vi "UHR-Fleezers Control (host) - 10.6.vi"() -> ()   [LabVIEW 2011] (continued)
              frame False {
              }
              frame True {
                n360 = property on="Sample Channel\nFlow" class="Bool (strict)"("Val(Sgnl)"=TRUE ("Stage Moving")) -> ()  [unwired: 2 in, 2 out]
              }
            }
            n361 = local write "Fl. Triggered..."(w574) -> ()
            n362 = local write "Tether"(w574) -> ()
            n363 = property on="Green Laser ON/Interlacing" class="Bool (strict)"("Val(Sgnl)"=w574) -> ()  [unwired: 2 in, 2 out]
            n364 = property on="Trap Pos. FB ON" class="Bool (strict)"("Val(Sgnl)"=w574) -> ()  [unwired: 2 in, 2 out]
            n365 = property on="Trap Trig. Fl." class="Bool (strict)"("Val(Sgnl)"=w574) -> ()  [unwired: 2 in, 2 out]
            n366 = property on="Dip for Protein" class="Bool (strict)"("Val(Sgnl)"=w574) -> ()  [unwired: 2 in, 2 out]
            n367 = property on="Pause dwell" class="Bool (strict)"("Val(Sgnl)"=w574) -> ()  [unwired: 2 in, 2 out]
          }
          frame #2 {
            n368 = property on="Trap Pos. FB Offset Factor" class="DigNum (strict)"("Val(Sgnl)"=i64 0 ("Value (Signaling)")) -> ()  [unwired: 2 in, 2 out]
          }
          frame #3 {
            n369 = local read "Saved Stage Positions"() -> (w583:dbl[][])
            n370 = local write "Stage Moving"(TRUE ("Stage Moving")) -> ()
            n371 = Array Subset(array=w583, index (row)=3 ("index"), length (row)=1 ("length"), index (col)=1 ("index"), length (col)=3 ("length")) -> (w588:dbl[][])
            n372 = Reshape Array(w588, 3 ("dimension size")) -> (w586:dbl[])
            n373 = Array To Cluster(array=w586) -> (cluster=w585:cluster{"[0]":dbl, "[1]":dbl, "[2]":dbl})
            n374 = call "Set Stage Position.vi"("Position"=w585, "error in"=w581, "VISA resource name in"=w582) -> ()  [unwired: 3 out]
          }
          frame #4 {
            w593 = FALSE ("Value (Signaling)")
            n375 = case shown="True" w592 {
              frame False {
              }
              frame True {
                n376 = property on="Sample Channel\nFlow" class="Bool (strict)"("Val(Sgnl)"=FALSE ("Stage Moving")) -> ()  [unwired: 2 in, 2 out]
              }
            }
            n377 = property on="Trap 1 (ON/OFF)" class="Bool (strict)"("Val(Sgnl)"=w593) -> ()  [unwired: 2 in, 2 out]
            n378 = property on="Trap 2 (ON/OFF)" class="Bool (strict)"("Val(Sgnl)"=w593) -> ()  [unwired: 2 in, 2 out]
            n379 = call <vilib>:"Beep.vi"() -> ()  [unwired: 3 in, 9 out]
          }
          frame #5 {
            n380 = property on="Move Cap. 2 (ADig Top)" class="Bool (strict)"("Val(Sgnl)"=TRUE ("Value (Signaling)")) -> ()  [unwired: 2 in, 2 out]
            n381 = property on="Tab Control" class="TabCtl (strict)"("Val(Sgnl)"=T4."Status" ("Value (Signaling)")) -> ()  [unwired: 2 in, 2 out]
          }
        }
      }
      event "Dip for Protein": Value Change {
        n382 = event-data() -> ()  [unwired: 1 in, 5 out]
        n383 = case shown="True" "Dip for Protein" {
          tunnel: w599 -> [_ w601]
          tunnel: w598 -> [_ w600]
          frame False {
          }
          frame True {
            n384 = while {
              tunnel: w601 -> [w612]
              tunnel: w600 -> [w611]
              i -> [w606]
              stop <- w608 stop-if-true
              n385 = Increment(x=w606) -> (x+1=→"Dip #":i32)
              n386 = flat-sequence {
                tunnel: w611 -> [w623]
                tunnel: w612 -> [w624]
                tunnel: [w624] -> w616
                tunnel: [w623] -> w615
                tunnel: [w617] -> w602
                tunnel: [w629] -> w610
                tunnel: [w630] -> w609
                tunnel: w616 -> [w631]
                tunnel: w615 -> [w632]
                tunnel: [w627] -> w603
                tunnel: w602 -> [w627]
                tunnel: [w640] -> w614
                tunnel: w610 -> [w640]
                tunnel: [w639] -> w613
                tunnel: w609 -> [w639]
                tunnel: [w636] -> w607
                tunnel: [w635] -> w604
                tunnel: w603 -> [w635]
                tunnel: w613 -> [w660]
                tunnel: w614 -> [w661]
                tunnel: w607 -> [w662]
                tunnel: w604 -> [w659]
                tunnel: [w718] -> w608
                frame #0 {
                  n387 = local read "Trap Pos. FB ON"() -> (w617:bool)
                  n388 = Compound Arithmetic op=AND("Flow ON\nduring dip?", "FB OFF when \nflow ON", w617) -> (w618:bool)
                  n389 = case shown="True" "Move trap \nbefore dip move?" {
                    frame False {
                    }
                    frame True {
                      n390 = property on="Trap Delta (MHz)" class="DigNum (strict)"("Val(Sgnl)"="Dipping Delta (MHz)") -> ()  [unwired: 2 in, 2 out]
                    }
                  }
                  n391 = property on="Green Laser ON/Interlacing" class="Bool (strict)"("Val(Sgnl)"="Green ON\nbefore dip?") -> ()  [unwired: 2 in, 2 out]
                  n392 = property on="Sample Channel\nFlow" class="Bool (strict)"("Val(Sgnl)"="Flow ON\nduring dip?") -> ()  [unwired: 2 in, 2 out]
                  n393 = case shown="True" w618 {
                    frame False {
                    }
                    frame True {
                      n394 = property on="Trap Pos. FB ON" class="Bool (strict)"("Val(Sgnl)"=FALSE ("Value (Signaling)")) -> ()  [unwired: 2 in, 2 out]
                    }
                  }
                }
                frame #1 {
                  n395 = local read "Saved Stage Positions"() -> (w634:dbl[][])
                  n396 = local write "Cancel dwell"(FALSE ("Cancel dwell")) -> ()
                  n397 = call "move to saved stage position.vi"("error in"=w632, "Stage VISA resource name in"=w631, "Position"="Dip Stage \nPosition", "Saved Stage Positions"=w634) -> ("VISA resource name out"=w629:refnum<visa-resource-name>, "error out"=w630:errorcluster)
                }
                frame #2 {
                  n398 = node-c288() -> (w638:T21)  [unwired: 4 in]
                  n399 = timed-loop {
                    timing: w638 -> [_]
                    timing-out: [_] -> w637
                    tunnel: [w644] -> w636
                    i -> [w641]
                    stop <- w645 stop-if-true
                    n400 = node-c288() -> ()  [unwired: 1 in, 1 out]
                    n401 = Greater Or Equal?(x=w641, y="Dip Duration (s)") -> (x >= y?=w653:bool)
                    n402 = local read "Dip for Protein"() -> (w646:bool)
                    n403 = local read "Dump Beads"() -> (w643:bool)
                    n404 = local read "Cancel dwell"() -> (w652:bool)
                    n405 = local read "Pause dwell"() -> (w649:bool)
                    n406 = Not(x=w646) -> (.not. x?=w651:bool)
                    n407 = Compound Arithmetic op=OR(w652, w653, w651) -> (w650:bool)
                    n408 = Select(t=FALSE, s=w649, f=w650) -> (s? t:f=w647:bool)
                    n409 = Not(x=w643) -> (.not. x?=w642:bool)
                    n410 = node-c288() -> ()  [unwired: 1 in, 1 out]
                    n411 = And(x=w646, y=w642) -> (x .and. y?=w644:bool)
                    n412 = Or(x=w647, y=w643) -> (x .or. y?=w645:bool)
                    "Dip Time (s)" <- w641
                  }
                  n413 = node-c288(w637) -> ()  [unwired: 1 out]
                }
                frame #3 {
                  n414 = case shown="True" w662 {
                    tunnel: w661 -> [_ w667]
                    tunnel: w660 -> [_ w666]
                    tunnel: w659 -> [_ w663]
                    frame False {
                    }
                    frame True {
                      n415 = flat-sequence {
                        tunnel: w666 -> [w671]
                        tunnel: w667 -> [w672]
                        tunnel: [w672] -> w665
                        tunnel: [w671] -> w664
                        tunnel: w663 -> [w668]
                        tunnel: w665 -> [w682]
                        tunnel: w664 -> [w681]
                        tunnel: w663 -> [w690]
                        frame #0 {
                          n416 = local read "Sample Channel\nFlow"() -> (w670:bool)
                          n417 = case shown="False" w670 {
                            tunnel: "Flow ON \nduring return\nfrom dip?" -> [w673 w676]
                            tunnel: w668 -> [_ w675]
                            frame False {
                              n418 = case shown="True" w673 {
                                frame False {
                                }
                                frame True {
                                n419 = property on="Sample Channel\nFlow" class="Bool (strict)"("Val(Sgnl)"=TRUE ("Value (Signaling)")) -> ()  [unwired: 2 in, 2 out]
                                }
                              }
                            }
                            frame True {
                              n420 = case shown="False" w676 {
                                tunnel: w675 -> [w677 _]
                                frame False {
                                n421 = property on="Trap Pos. FB ON" class="Bool (strict)"("Val(Sgnl)"=w677) -> ()  [unwired: 2 in, 2 out]
                                n422 = property on="Sample Channel\nFlow" class="Bool (strict)"("Val(Sgnl)"=FALSE ("Value (Signaling)")) -> ()  [unwired: 2 in, 2 out]
                                }
                                frame True {
                                }
                              }
                            }
                          }
                        }
                        frame #1 {
                          # "For turning on green laser before stage reaches lower spot"
                          n423 = case shown="True" "Green ON\nafter start\nreturn?" {
                            frame False {
                            }
                            frame True {
                              n424 = flat-sequence {
                                frame #0 {
                                n425 = Multiply(x="Green delay after \nstart return (s)", y=1000.0) -> (x*y=w687:dbl)
                                n426 = Wait (ms)(milliseconds to wait=w687) -> ()  [unwired: 1 out]
                                }
                                frame #1 {
                                n427 = property on="Green Laser ON/Interlacing" class="Bool (strict)"("Val(Sgnl)"=TRUE ("Value (Signaling)")) -> ()  [unwired: 2 in, 2 out]
                                }
                              }
                            }
                          }
                          n428 = local read "Saved Stage Positions"() -> (w685:dbl[][])
                          n429 = local write "Cancel dwell"(FALSE ("Cancel dwell")) -> ()
                          n430 = call "move to saved stage position.vi"("error in"=w681, "Stage VISA resource name in"=w682, "Position"="Return Stage \nPosition", "Saved Stage Positions"=w685) -> ("error out"=w683:errorcluster)  [unwired: 1 out]
                          n431 = local write "Stage Control Serial Error"(w683) -> ()
                        }
                        frame #2 {
                          n432 = property on="Trap Pos. FB ON" class="Bool (strict)"("Val(Sgnl)"=w690) -> ()  [unwired: 2 in, 2 out]
                          n433 = case shown="True" "Green ON \nafter return?" {
                            frame False {
                            }
                            frame True {
                              n434 = property on="Green Laser ON/Interlacing" class="Bool (strict)"("Val(Sgnl)"=TRUE ("Value (Signaling)")) -> ()  [unwired: 2 in, 2 out]
                            }
                          }
                          n435 = case shown="True" "Move trap after return?" {
                            frame False {
                            }
                            frame True {
                              n436 = property on="Trap Delta (MHz)" class="DigNum (strict)"("Val(Sgnl)"="Dip Trap Delta 2 (MHz)") -> ()  [unwired: 2 in, 2 out]
                            }
                          }
                          n437 = case shown="True" "Save data after return?" {
                            frame False {
                            }
                            frame True {
                              n438 = property on="Start Saving" class="Bool (strict)"("Val(Sgnl)"=TRUE ("Value (Signaling)")) -> ()  [unwired: 2 in, 2 out]
                            }
                          }
                          n439 = property on="Sample Channel\nFlow" class="Bool (strict)"("Val(Sgnl)"="Flow ON\nduring daq?") -> ()  [unwired: 2 in, 2 out]
                        }
                        frame #3 {
                          n440 = node-c288() -> (w699:T21)  [unwired: 4 in]
                          n441 = timed-loop {
                            timing: w699 -> [_]
                            timing-out: [_] -> w698
                            i -> [w700]
                            stop <- w702 stop-if-true
                            n442 = node-c288() -> ()  [unwired: 1 in, 1 out]
                            n443 = local read "Dump Beads"() -> (w701:bool)
                            n444 = Greater Or Equal?(x=w700, y="Dwell Duration (s)") -> (x >= y?=w707:bool)
                            n445 = local read "Dip for Protein"() -> (w704:bool)
                            n446 = Not(x=w704) -> (.not. x?=w703:bool)
                            n447 = Compound Arithmetic op=OR(w707, "Cancel dwell", w703) -> (w706:bool)
                            n448 = node-c288() -> ()  [unwired: 1 in, 1 out]
                            n449 = Select(t=FALSE, s="Pause dwell", f=w706) -> (s? t:f=w709:bool)
                            n450 = Or(x=w709, y=w701) -> (x .or. y?=w702:bool)
                            "Dwell Time (s)" <- w700
                          }
                          n451 = node-c288(w698) -> ()  [unwired: 1 out]
                        }
                      }
                    }
                  }
                }
                frame #4 {
                  n452 = local read "Dip for Protein"() -> (w719:bool)
                  n453 = local read "Dump Beads"() -> (w716:bool)
                  n454 = local write "Cancel dwell"(FALSE ("Cancel dwell")) -> ()
                  n455 = Not(x=w719) -> (.not. x?=w720:bool)
                  n456 = Not(x="Cont. Repeat Dipping?") -> (.not. x?=w722:bool)
                  n457 = Compound Arithmetic op=OR(w720, w722, w716) -> (w718:bool)
                }
              }
            }
          }
        }
      }
      event "Profile": Value Change {
        n458 = event-data() -> ()  [unwired: 1 in, 5 out]
        n459 = flat-sequence {
          tunnel: w731 -> [w734]
          tunnel: w730 -> [w742]
          tunnel: [w736] -> w729
          tunnel: [w735] -> w728
          tunnel: [w733] -> w726
          tunnel: [w732] -> w723
          tunnel: w729 -> [w749]
          tunnel: w728 -> [w748]
          tunnel: [w746] -> w727
          tunnel: w726 -> [w747]
          tunnel: [w745] -> w725
          tunnel: [w744] -> w724
          tunnel: w723 -> [w744]
          tunnel: w727 -> [w753]
          tunnel: w725 -> [w752]
          tunnel: w724 -> [w751]
          frame #0 {
            n460 = call "Read Stage Position.vi"("error in"=w742, "VISA resource name in"=w734) -> ("Current Position"=w732:cluster{dbl, dbl, dbl}, "error out"=w735:errorcluster, "VISA resource name out"=w733:refnum<visa-resource-name>)  [unwired: 1 out]
            "Current Position" <- w732
            n461 = local write "Stage Control Serial Error"(w735) -> ()
            n462 = Unbundle(w732) -> (w739:dbl, w741:dbl, w737:dbl)
            n463 = Add(x=w741, y="Y change (mm)") -> (x+y=w738:dbl)
            n464 = Bundle(w739, w738, w737) -> (w736:cluster{dbl, dbl, dbl})  [unwired: 1 in]
          }
          frame #1 {
            # "move to new position and start saving"
            n465 = local write "Stage Moving"(TRUE ("Stage Moving")) -> ()
            n466 = local write "Start Saving"(TRUE ("Start Saving")) -> ()
            n467 = call "Set Stage Position.vi"("Position"=w749, "error in"=w748, "VISA resource name in"=w747) -> ("error out"=w745:errorcluster, "VISA resource name out"=w746:refnum<visa-resource-name>)  [unwired: 1 out]
          }
          frame #2 {
            # "go back to start"
            n468 = call "Set Stage Position.vi"("Position"=w751, "error in"=w752, "VISA resource name in"=w753) -> ()  [unwired: 3 out]
          }
          frame #3 {
            # "stop saving"
            n469 = local write "Stop Saving"(TRUE ("Stop Saving")) -> ()
            n470 = local write "Stage Moving"(FALSE ("Stage Moving")) -> ()
          }
        }
      }
      event "Move to Position 1", "Move to Position 2", "Move to Position 3", "Move to Position 4", "Move to Position 5", "Lower Ch. Cap.": Value Change {
        n471 = event-data() -> ()  [unwired: 1 in, 5 out]
        n472 = Or(x="Move to Position 5", y="Lower Ch. Cap.") -> (x .or. y?=w759:bool)
        n473 = Build Array("Move to Position 1", "Move to Position 2", "Move to Position 3", "Move to Position 4", w759) -> (w762:bool[])
        n474 = Boolean Array To Number(Boolean array=w762) -> (number=w761:u32)
        n475 = Logarithm Base 2(1:w761) -> (0:w760:dbl)
        n476 = flat-sequence {
          tunnel: w760 -> [w771]
          tunnel: w757 -> [w769]
          tunnel: w756 -> [w768]
          frame #0 {
            n477 = local read "Saved Stage Positions"() -> (w779:dbl[][])
            n478 = Array Subset(array=w779, index (row)=w771, length (row)=1 ("length"), index (col)=1 ("index"), length (col)=3 ("length")) -> (w776:dbl[][])
            n479 = Reshape Array(w776, 3 ("dimension size")) -> (w774:dbl[])
            n480 = Array To Cluster(array=w774) -> (cluster=w773:cluster{"[0]":dbl, "[1]":dbl, "[2]":dbl})
            n481 = call "Set Stage Position.vi"("Position"=w773, "error in"=w768, "VISA resource name in"=w769) -> ("error out"=w772:errorcluster)  [unwired: 2 out]
            n482 = local write "Stage Moving"(TRUE ("Stage Moving")) -> ()
            n483 = local write "Stage Control Serial Error"(w772) -> ()
          }
          frame #1 {
            n484 = local write "Stage Moving"(FALSE ("Stage Moving")) -> ()
            n485 = call <vilib>:"Beep.vi"() -> ()  [unwired: 3 in, 9 out]
          }
        }
      }
      event "Got ADig bead": Value Change {
        n486 = event-data() -> ()  [unwired: 1 in, 5 out]
        n487 = flat-sequence {
          frame #0 {
            n488 = local read "Cap 1 Samp Flow ON"() -> (w783:bool)
            n489 = case shown="True" w783 {
              frame False {
              }
              frame True {
                n490 = property on="Sample Channel\nFlow" class="Bool (strict)"("Val(Sgnl)"=TRUE ("Value (Signaling)")) -> ()  [unwired: 2 in, 2 out]
              }
            }
          }
          frame #1 {
            n491 = property on="Inject Pump 3" class="Bool (strict)"("Val(Sgnl)"=FALSE ("Value (Signaling)")) -> ()  [unwired: 2 in, 2 out]
          }
          frame #2 {
            n492 = property on="Move Cap. 1 (DNA Bottom)" class="Bool (strict)"("Val(Sgnl)"=TRUE ("Value (Signaling)")) -> ()  [unwired: 2 in, 2 out]
          }
        }
      }
      event "Force FB Data\nScript": Value Change {
        n493 = event-data() -> ()  [unwired: 1 in, 5 out]
        n494 = flat-sequence {
          tunnel: w792 -> [w796]
          tunnel: w793 -> [w797]
          tunnel: [w797] -> w788
          tunnel: [w796] -> w787
          tunnel: w788 -> [w800]
          tunnel: w787 -> [w799]
          tunnel: ["Trap Trig Fl."] -> w789
          tunnel: [w825] -> w790
          tunnel: w789 -> [w825]
          tunnel: [w829] -> w791
          tunnel: w790 -> [w829]
          tunnel: w791 -> [w831]
          frame #0 {
            n495 = property on="Trap Delta (MHz)" class="DigNum (strict)"("Val(Sgnl)"="Trap Delta Before Moving") -> ()  [unwired: 2 in, 2 out]
          }
          frame #1 {
            n496 = local read "Saved Stage Positions"() -> (w802:dbl[][])
            n497 = local write "FB Trap Pos Offset"(0.0 ("FB Trap Pos Offset")) -> ()
            n498 = property on="Trap Pos. FB Offset Factor" class="DigNum (strict)"("Val(Sgnl)"=i64 0 ("Value (Signaling)")) -> ()  [unwired: 2 in, 2 out]
            n499 = local write "Stage Moving"(TRUE ("Stage Moving")) -> ()
            n500 = call "move to saved stage position.vi"("error in"=w799, "Stage VISA resource name in"=w800, "Position"="Stage Position To Establish FB", "Saved Stage Positions"=w802) -> ("error out"=w798:errorcluster)  [unwired: 1 out]
            n501 = local write "Stage Control Serial Error"(w798) -> ()
          }
          frame #2 {
            n502 = call <vilib>:"Beep.vi"() -> ()  [unwired: 3 in, 9 out]
            n503 = Multiply(x="Wait (s)", y=u32 1000 ("milliseconds to wait")) -> (x*y=w808:u32)
            n504 = property on="Trap Delta (MHz)" class="DigNum (strict)"("Val(Sgnl)"="Starting \nTrap Delta (MHz)") -> ()  [unwired: 2 in, 2 out]
            n505 = local write "Stage Moving"(FALSE ("Stage Moving")) -> ()
            n506 = Wait (ms)(milliseconds to wait=w808) -> ()  [unwired: 1 out]
            n507 = property on="Tab Control 2" class="TabCtl (strict)"("Val(Sgnl)"=T6."Feedback on Trap Position" ("Value (Signaling)")) -> ()  [unwired: 2 in, 2 out]
            n508 = property on="Tab Control" class="TabCtl (strict)"("Val(Sgnl)"=T4."Trap Control (RF)" ("Value (Signaling)")) -> ()  [unwired: 2 in, 2 out]
          }
          frame #3 {
            n509 = property on="Set Reading to\nSetpoint" class="Bool (strict)"("Val(Sgnl)"=TRUE ("Value (Signaling)")) -> ()  [unwired: 2 in, 2 out]
            n510 = Wait (ms)(milliseconds to wait=u32 500) -> ()  [unwired: 1 out]
          }
          frame #4 {
            n511 = property on="Trap Pos. FB ON" class="Bool (strict)"("Val(Sgnl)"=TRUE ("Value (Signaling)")) -> ()  [unwired: 2 in, 2 out]
            n512 = Wait (ms)(milliseconds to wait=u32 250) -> ()  [unwired: 1 out]
          }
          frame #5 {
            n513 = case shown="False" "Trap Trig Fl." {
              frame False {
                n514 = case shown="True" "Green ON after FB ON?" {
                  selector: "Green ON after FB ON?" -> [_ w824]
                  frame False {
                  }
                  frame True {
                    n515 = property on="Green Laser ON/Interlacing" class="Bool (strict)"("Val(Sgnl)"=w824) -> ()  [unwired: 2 in, 2 out]
                  }
                }
              }
              frame True {
              }
            }
            n516 = case shown="True" "Remove Action Offset" {
              tunnel: TRUE ("Value (Signaling)") -> [w821 w822]
              frame False {
                n517 = property on="Remove Unwinding Offset" class="Bool (strict)"("Val(Sgnl)"=w821) -> ()  [unwired: 2 in, 2 out]
              }
              frame True {
                n518 = property on="Remove Action Offset" class="Bool (strict)"("Val(Sgnl)"=w822) -> ()  [unwired: 2 in, 2 out]
              }
            }
            n519 = Wait (ms)(milliseconds to wait=u32 250) -> ()  [unwired: 1 out]
          }
          frame #6 {
            n520 = property on="Start Saving" class="Bool (strict)"("Val(Sgnl)"=TRUE ("Value (Signaling)")) -> ()  [unwired: 2 in, 2 out]
            n521 = Wait (ms)(milliseconds to wait=u32 5000) -> ()  [unwired: 1 out]
          }
          frame #7 {
            w828 = TRUE ("Value (Signaling)")
            n522 = property on="Rem fb disp offset" class="Bool (strict)"("Val(Sgnl)"=w828) -> ()  [unwired: 2 in, 2 out]
            n523 = property on="Remove Offset" class="Bool (strict)"("Val(Sgnl)"=w828) -> ()  [unwired: 2 in, 2 out]
            n524 = Wait (ms)(milliseconds to wait=u32 100) -> ()  [unwired: 1 out]
          }
          frame #8 {
            n525 = case shown="True" w831 {
              frame False {
              }
              frame True {
                n526 = local write "Trap Trig. Fl."(TRUE ("Value (Signaling)")) -> ()
              }
            }
          }
          frame #9 {
            n527 = case shown="True" "Start dipping after?" {
              frame False {
              }
              frame True {
                n528 = flat-sequence {
                  frame #0 {
                    n529 = Multiply(x="Delay before dipping (s)", y=1000.0) -> (x*y=w835:dbl)
                    n530 = Wait (ms)(milliseconds to wait=w835) -> ()  [unwired: 1 out]
                  }
                  frame #1 {
                    n531 = property on="Dip for Protein" class="Bool (strict)"("Val(Sgnl)"=TRUE ("Value (Signaling)")) -> ()  [unwired: 2 in, 2 out]
                    n532 = local write "Scripts"(T1."Dipping" ("Scripts")) -> ()
                  }
                }
              }
            }
          }
        }
      }
      event "Fixed Traps Data\nScript": Value Change {
        n533 = event-data() -> ()  [unwired: 1 in, 5 out]
        n534 = flat-sequence {
          frame #0 {
            n535 = case shown="True" "Green ON" {
              frame False {
              }
              frame True {
                n536 = property on="Green Laser ON/Interlacing" class="Bool (strict)"("Val(Sgnl)"=TRUE) -> ()  [unwired: 2 in, 2 out]
              }
            }
            n537 = local write "Offset (nm)"(0.0 ("Offset (nm)")) -> ()
            n538 = property on="Sample Channel\nFlow" class="Bool (strict)"("Val(Sgnl)"=FALSE ("Value (Signaling)")) -> ()  [unwired: 2 in, 2 out]
            n539 = property on="Trap Delta (MHz)" class="DigNum (strict)"("Val(Sgnl)"="Fixed Traps Trap Delta (MHz)") -> ()  [unwired: 2 in, 2 out]
          }
          frame #1 {
            n540 = Wait (ms)(milliseconds to wait=u32 1000) -> ()  [unwired: 1 out]
          }
          frame #2 {
            n541 = local write "Start Saving"(TRUE ("Start Saving")) -> ()
          }
          frame #3 {
            n542 = local read "Bead Sep. Int. Time (s)"() -> (w846:dbl)
            n543 = Multiply(x=w846, y=1000.0) -> (x*y=w848:dbl)
            n544 = Wait (ms)(milliseconds to wait=w848) -> ()  [unwired: 1 out]
          }
          frame #4 {
            n545 = property on="Remove Offset" class="Bool (strict)"("Val(Sgnl)"=TRUE ("Value (Signaling)")) -> ()  [unwired: 2 in, 2 out]
          }
          frame #5 {
            n546 = property on="Dip for Protein" class="Bool (strict)"("Val(Sgnl)"="Start dipping after?") -> ()  [unwired: 2 in, 2 out]
          }
        }
      }
      event "Got DNA bead": Value Change {
        n547 = event-data() -> ()  [unwired: 1 in, 5 out]
        n548 = flat-sequence {
          frame #0 {
            n549 = local read "Daq spot flow on"() -> (w853:bool)
            n550 = case shown="True" w853 {
              frame False {
              }
              frame True {
                n551 = property on="Sample Channel\nFlow" class="Bool (strict)"("Val(Sgnl)"=TRUE ("Value (Signaling)")) -> ()  [unwired: 2 in, 2 out]
              }
            }
            n552 = property on="Got DNA bead" class="Bool"("Key Focus"=FALSE) -> ()  [unwired: 2 in, 2 out]
          }
          frame #1 {
            n553 = property on="Inject Pump 1" class="Bool (strict)"("Val(Sgnl)"=FALSE ("Value (Signaling)")) -> ()  [unwired: 2 in, 2 out]
          }
          frame #2 {
            n554 = property on="Cal/Data Acq. Spot" class="Bool (strict)"("Val(Sgnl)"=TRUE ("Value (Signaling)")) -> ()  [unwired: 2 in, 2 out]
          }
        }
      }
      event "Take Stepping Data": Value Change {
        n555 = event-data() -> ()  [unwired: 1 in, 5 out]
        n556 = local read "Save ave N"() -> (w865:dbl)
        n557 = flat-sequence {
          tunnel: w865 -> [w867]
          tunnel: [w867] -> w860
          tunnel: [w869] -> w861
          tunnel: w860 -> [w869]
          tunnel: [w871] -> w862
          tunnel: w861 -> [w871]
          tunnel: [w874] -> w863
          tunnel: w862 -> [w874]
          tunnel: [w876] -> w864
          tunnel: w863 -> [w876]
          tunnel: [w878] -> w858
          tunnel: w864 -> [w878]
          tunnel: w858 -> [w881]
          tunnel: [w881] -> w857
          tunnel: w857 -> [w882]
          tunnel: [w882] -> w859
          tunnel: w859 -> [w888]
          frame #0 {
            n558 = property on="Save ave N" class="DigNum (strict)"("Val(Sgnl)"="Save ave factor") -> ()  [unwired: 2 in, 2 out]
          }
          frame #1 {
            n559 = Wait (ms)(milliseconds to wait=u32 100) -> ()  [unwired: 1 out]
          }
          frame #2 {
            n560 = local read "Offset 2 Start (MHz)"() -> (w873:dbl)
            n561 = property on="Saved AOD Raster Scan Parameter Sets" class="Arr (strict)"("Index Values"=u32[] [2]) -> ()  [unwired: 2 in, 2 out]
            n562 = property on="Trap Delta (MHz)" class="DigNum (strict)"("Val(Sgnl)"=w873) -> ()  [unwired: 2 in, 2 out]
          }
          frame #3 {
            n563 = property on="Load parameters" class="Bool (strict)"("Val(Sgnl)"=TRUE ("Value (Signaling)")) -> ()  [unwired: 2 in, 2 out]
          }
          frame #4 {
            n564 = Wait (ms)(milliseconds to wait=u32 100) -> ()  [unwired: 1 out]
          }
          frame #5 {
            n565 = property on="Trap Raster Scan" class="Bool (strict)"("Val(Sgnl)"=TRUE ("Value (Signaling)")) -> ()  [unwired: 2 in, 2 out]
          }
          frame #6 {
            n566 = Wait (ms)(milliseconds to wait=u32 1000) -> ()  [unwired: 1 out]
          }
          frame #7 {
            n567 = while {
              stop <- w885 stop-if-true
              n568 = local read "Raster Scanning..."() -> (w887:bool)
              n569 = local read "Saving..."() -> (w886:bool)
              n570 = Not(x=w886) -> (.not. x?=w883:bool)
              n571 = Not(x=w887) -> (.not. x?=w884:bool)
              n572 = And(x=w884, y=w883) -> (x .and. y?=w885:bool)
            }
          }
          frame #8 {
            n573 = property on="Save ave N" class="DigNum (strict)"("Val(Sgnl)"=w888) -> ()  [unwired: 2 in, 2 out]
          }
        }
      }
      event "Step Size (nm)": Value Change {
        n574 = event-data() -> ()  [unwired: 1 in, 5 out]
        n575 = flat-sequence {
          frame #0 {
            n576 = property on="Saved AOD Raster Scan Parameter Sets" class="Arr (strict)"("Index Values"=u32[] [1]) -> ()  [unwired: 2 in, 2 out]
          }
          frame #1 {
            n577 = Multiply(x="N Steps", y="Step Size (nm)") -> (x*y=w890:dbl)
            n578 = property on="Scan Speed AOD (nm/s) 2" class="DigNum (strict)"("Value"="Step Size (nm)") -> ()  [unwired: 2 in, 2 out]
            n579 = property on="Step Size AOD (nm) 2" class="DigNum (strict)"("Value"="Step Size (nm)") -> ()  [unwired: 2 in, 2 out]
            n580 = property on="Scan Range AOD (nm) 2" class="DigNum (strict)"("Value"=w890) -> ()  [unwired: 2 in, 2 out]
          }
        }
      }
      event "Take Detection Laser\nImage": Value Change {
        n581 = event-data() -> ()  [unwired: 1 in, 5 out]
        n582 = flat-sequence {
          tunnel: [w918] -> w908
          tunnel: [w917] -> w901
          tunnel: [w916] -> w893
          tunnel: [w921] -> w909
          tunnel: w908 -> [w921]
          tunnel: [w920] -> w902
          tunnel: w901 -> [w920]
          tunnel: [w919] -> w894
          tunnel: w893 -> [w919]
          tunnel: [w925] -> w910
          tunnel: w909 -> [w925]
          tunnel: [w924] -> w903
          tunnel: w902 -> [w924]
          tunnel: [w923] -> w895
          tunnel: w894 -> [w923]
          tunnel: [w931] -> w911
          tunnel: w910 -> [w931]
          tunnel: [w930] -> w904
          tunnel: w903 -> [w930]
          tunnel: [w929] -> w896
          tunnel: w895 -> [w929]
          tunnel: [w935] -> w912
          tunnel: w911 -> [w935]
          tunnel: [w934] -> w905
          tunnel: w904 -> [w934]
          tunnel: [w933] -> w897
          tunnel: w896 -> [w933]
          tunnel: [w939] -> w913
          tunnel: w912 -> [w939]
          tunnel: [w938] -> w906
          tunnel: w905 -> [w938]
          tunnel: [w937] -> w898
          tunnel: w897 -> [w937]
          tunnel: [w943] -> w914
          tunnel: w913 -> [w943]
          tunnel: [w942] -> w907
          tunnel: w906 -> [w942]
          tunnel: [w941] -> w899
          tunnel: w898 -> [w941]
          tunnel: w914 -> [w949]
          tunnel: w907 -> [w948]
          tunnel: [w946] -> w900
          tunnel: w899 -> [w946]
          tunnel: w900 -> [w950]
          frame #0 {
            n583 = local read "Green Laser ON/Interlacing"() -> (w918:bool)
            n584 = local read "Green laser mode"() -> (w917:enum32{"Laser ON", "Laser OFF", "Interlace"})
            n585 = local read "Green FB On/Off"() -> (w916:bool)
          }
          frame #1 {
            n586 = property on="Green FB On/Off" class="Bool (strict)"("Val(Sgnl)"=FALSE ("Value (Signaling)")) -> ()  [unwired: 2 in, 2 out]
          }
          frame #2 {
            n587 = property on="Green Laser ON/Interlacing" class="Bool (strict)"("Val(Sgnl)"=TRUE ("Value (Signaling)")) -> ()  [unwired: 2 in, 2 out]
            n588 = property on="Flip Green Filter" class="Bool (strict)"("Val(Sgnl)"=TRUE ("Value (Signaling)")) -> ()  [unwired: 2 in, 2 out]
            n589 = property on="Green laser mode" class="RadioBtnsControl (strict)"("Val(Sgnl)"=enum32{"Laser ON", "Laser OFF", "Interlace"}."Laser ON" ("Value (Signaling)")) -> ()  [unwired: 2 in, 2 out]
          }
          frame #3 {
            n590 = Wait (ms)(milliseconds to wait=u32 500) -> ()  [unwired: 1 out]
          }
          frame #4 {
            n591 = property on="Confocal Image" class="Bool (strict)"("Val(Sgnl)"=TRUE ("Value (Signaling)")) -> ()  [unwired: 2 in, 2 out]
          }
          frame #5 {
            n592 = Wait (ms)(milliseconds to wait=u32 2000) -> ()  [unwired: 1 out]
          }
          frame #6 {
            n593 = while {
              stop <- w944 stop-if-true
              n594 = local read "Saving..."() -> (w945:bool)
              n595 = Not(x=w945) -> (.not. x?=w944:bool)
            }
          }
          frame #7 {
            n596 = property on="Flip Green Filter" class="Bool (strict)"("Val(Sgnl)"=TRUE ("Value (Signaling)")) -> ()  [unwired: 2 in, 2 out]
            n597 = property on="Green Laser ON/Interlacing" class="Bool (strict)"("Val(Sgnl)"=w949) -> ()  [unwired: 2 in, 2 out]
            n598 = property on="Green laser mode" class="RadioBtnsControl (strict)"("Val(Sgnl)"=w948) -> ()  [unwired: 2 in, 2 out]
          }
          frame #8 {
            n599 = property on="Green FB On/Off" class="Bool (strict)"("Val(Sgnl)"=w950) -> ()  [unwired: 2 in, 2 out]
          }
        }
      }
      event "Stop All": Value Change {
        n600 = event-data() -> ()  [unwired: 1 in, 5 out]
        n601 = local read "Stop All"() -> (w951:bool)
      }
    }
    n602 = node-c288() -> ()  [unwired: 1 in, 1 out]
  }
  n603 = disable-structure shown="Disabled" {
    disable-tunnel: [w953 _] -> w230
    disable-tunnel: w50 -> [w952 _]
    frame Disabled {
      n604 = node-c288() -> (w955:T21)  [unwired: 4 out]
      n605 = timed-loop "Rough control of MCL mirror stage (debugging)" {
        tunnel: w952 -> [w958]
        tunnel: [w957] -> w953
        timing: w955 -> [_]
        timing-out: [_] -> w954
        stop <- w957 stop-if-true
        n606 = node-c288() -> ()  [unwired: 2 out]
        n607 = case shown="1" "MCL Mode" {
          tunnel: w958 -> [_ w961 w1008]
          frame 0, Default {
          }
          frame 1 {
            n608 = node-c288() -> (w963:T21)  [unwired: 4 out]
            n609 = timed-loop "Oscillate MCL mirror" {
              timing: w963 -> [_]
              timing-out: [_] -> w962
              tunnel: w961 -> [w1002]
              i -> [w1001]
              stop <- w964 stop-if-true
              n610 = node-c288() -> (w1000:i64)  [unwired: 1 out]
              n611 = Multiply(x="AO1", y=32767.0) -> (x*y=w996:dbl)
              n612 = Multiply(x="AO2", y=32767.0) -> (x*y=w991:dbl)
              n613 = Divide(x=w996, y=10.0) -> (x/y=w997:dbl)
              n614 = Divide(x=w991, y=10.0) -> (x/y=w992:dbl)
              n615 = To Word Integer(number=w997) -> (16bit integer=w989:i16)
              n616 = To Word Integer(number=w992) -> (16bit integer=w988:i16)
              n617 = Divide(x=w1000, y=i64 1000) -> (x/y=w971:dbl)
              n618 = Multiply(x=w971, y=w1001) -> (x*y=w982:dbl)
              n619 = Multiply(x="Osc. freq. (Hz) 2", y=6.283185307179586) -> (x*y=w983:dbl)
              n620 = Multiply(x=w983, y=w982) -> (x*y=w981:dbl)
              n621 = Sine(x=w981) -> (sin(x)=w980:dbl)
              n622 = Multiply(x=w980, y="Osc. amp. (V)") -> (x*y=w978:dbl)
              n623 = Add(x=w978, y="Osc. center (V)") -> (x+y=w976:dbl)
              n624 = Divide(x=w976, y=10.0) -> (x/y=w974:dbl)
              n625 = Multiply(x=w974, y=32767.0) -> (x*y=w969:dbl)
              n626 = Select(t=w969, s="Scan axis", f=w989) -> (s? t:f=w987:dbl)
              n627 = Select(t=w988, s="Scan axis", f=w969) -> (s? t:f=w986:dbl)
              n628 = local read "MCL Mode"() -> (w968:u16)
              n629 = Not Equal?(x=w968, y=u16 1) -> (x != y?=w965:bool)
              n630 = local read "Stop All"() -> (w966:bool)
              n631 = xnode "Read/Write Control"("FPGA VI Reference In"=w1002, "AO1"=w987, "AO2"=w986) -> ()  [unwired: 1 in, 2 out]
              n632 = Compound Arithmetic op=OR(w966, w965) -> (w964:bool)
              n633 = node-c288() -> ()  [unwired: 2 out]
            }
            n634 = node-c288(w962) -> ()  [unwired: 1 out]
          }
          frame 2 {
            n635 = case shown="True" "Start Scan" {
              tunnel: w1008 -> [_ w1020]
              frame False {
              }
              frame True {
                n636 = Subtract(x="End (V)", y="Begin (V)") -> (x-y=w1016:dbl)
                n637 = Decrement(x="N Points") -> (x-1=w1015:dbl)
                n638 = Divide(x=w1016, y=w1015) -> (x/y=w1013:dbl)
                n639 = for {
                  N: "N Points" -> [_]
                  tunnel: "Begin (V)" -> [w1033]
                  tunnel: w1020 -> [w1025]
                  tunnel: [w1024] -> w1019 mode=indexing
                  tunnel: w1013 -> [w1023]
                  tunnel: [w1021] -> w1012 mode=indexing
                  i -> [w1032]
                  n640 = Multiply(x=w1023, y=w1032) -> (x*y=w1031:dbl)
                  n641 = Add(x=w1033, y=w1031) -> (x+y=w1028:dbl)
                  n642 = local read "Scan axis"() -> (w1022:bool)
                  n643 = local read "AO1"() -> (w1030:dbl)
                  n644 = local read "AO2"() -> (w1029:dbl)
                  n645 = Select(t=w1028, s=w1022, f=w1030) -> (s? t:f=w1027:dbl)
                  n646 = Select(t=w1029, s=w1022, f=w1028) -> (s? t:f=w1026:dbl)
                  n647 = flat-sequence {
                    tunnel: w1027 -> [w1037]
                    tunnel: w1026 -> [w1036]
                    tunnel: w1025 -> [w1034]
                    tunnel: [w1047] -> w1024
                    tunnel: [w1046] -> w1021
                    frame #0 {
                      w1040 = 10.0 ("y")
                      w1035 = 32767.0 ("y")
                      n648 = Multiply(x=w1037, y=w1035) -> (x*y=w1043:dbl)
                      n649 = Multiply(x=w1036, y=w1035) -> (x*y=w1041:dbl)
                      n650 = Divide(x=w1043, y=w1040) -> (x/y=w1044:dbl)
                      n651 = Divide(x=w1041, y=w1040) -> (x/y=w1042:dbl)
                      n652 = To Word Integer(number=w1044) -> (16bit integer=w1038:i16)
                      n653 = To Word Integer(number=w1042) -> (16bit integer=w1039:i16)
                      n654 = xnode "Read/Write Control"("FPGA VI Reference In"=w1034, "AO1"=w1038, "AO2"=w1039) -> ()  [unwired: 1 in, 2 out]
                    }
                    frame #1 {
                      n655 = Wait (ms)(milliseconds to wait="DAQ Delay (ms)") -> ()  [unwired: 1 out]
                    }
                    frame #2 {
                      n656 = local read "Slow mean"() -> (w1047:dbl)
                      n657 = local read "Sigma"() -> (w1046:dbl)
                    }
                  }
                }
                n658 = Bundle("Begin (V)"="Begin (V)", w1013, w1019) -> (→"MCL Scan":cluster{"Begin (V)":dbl, dbl, dbl[]})  [unwired: 1 out]
                n659 = Bundle("Begin (V)"="Begin (V)", w1013, w1012) -> (→"MCL Scan 2":cluster{"Begin (V)":dbl, dbl, dbl[]})  [unwired: 1 out]
              }
            }
          }
        }
        n660 = local read "Stop All"() -> (w957:bool)
        n661 = node-c288() -> ()  [unwired: 2 out]
      }
      n662 = node-c288(w954) -> ()  [unwired: 1 out]
    }
    frame Enabled {
    }
  }
  n663 = node-c288(3 ("Processor")) -> (w90:T21)  [unwired: 3 out]
  n664 = node-c288(2 ("Processor")) -> (w92:T21)  [unwired: 3 out]
  n665 = node-c288() -> (w94:T21)  [unwired: 4 out]
  n666 = timed-loop "Oscillate Trap/AOM (fishing, debugging)" {
    tunnel: w50 -> [w1051]
    tunnel: [w1050] -> w95
    timing: w90 -> [_]
    timing-out: [_] -> w89
    stop <- w1050 stop-if-true
    n667 = node-c288() -> ()  [unwired: 2 out]
    n668 = event shown="[0] \"Oscillate Set 1\", \"Fish for Tether\": Value Change" {
      selector: _ -> [_ _ _]
      dyn-events: _ -> [_ _ _]
      timeout: _ -> [_ _ _]
      tunnel: w1051 -> [w1058 _ _]
      tunnel: [FALSE ("Stop All") _ w1343] -> w1050
      event "Oscillate Set 1", "Fish for Tether": Value Change {
        n669 = event-data() -> ()  [unwired: 6 out]
        n670 = local read "Oscillate Set 1"() -> (w1057:bool)
        n671 = Or(x=w1057, y="Fish for Tether") -> (x .or. y?=w1055:bool)
        n672 = case shown="True" w1055 {
          tunnel: w1058 -> [_ w1061]
          tunnel: "Fish for Tether" -> [_ w1060]
          frame False {
          }
          frame True {
            n673 = case shown="True" w1060 {
              selector: w1060 -> [w1064 w1070]
              tunnel: [w1064 w1070] -> w1059
              frame False {
              }
              frame True {
                n674 = local write "Scan axis 2"(TRUE) -> ()
                n675 = local write "Tether"(FALSE ("Tether")) -> ()
                n676 = local read "Flow ON during cal?"() -> (w1065:bool)
                n677 = property on="Trap Delta (MHz)" class="DigNum (strict)"("Val(Sgnl)"="Furthest Delta (MHz)") -> ()  [unwired: 2 in, 2 out]
                n678 = Or(x="Flow ON during \nfishing?", y=w1065) -> (x .or. y?=w1066:bool)
                n679 = Wait (ms)(milliseconds to wait=u32 500) -> ()  [unwired: 1 out]
                n680 = property on="Sample Channel\nFlow" class="Bool (strict)"("Val(Sgnl)"=w1066) -> ()  [unwired: 2 in, 2 out]
              }
            }
            n681 = node-c288() -> (w1063:T21)  [unwired: 4 out]
            n682 = timed-loop "Oscillate AOD" {
              timing: w1063 -> [_]
              timing-out: [_] -> w1062
              tunnel: w1061 -> [w1080]
              tunnel: w1059 -> [w1073]
              i -> [w1082]
              stop <- w1079 stop-if-true
              n683 = node-c288() -> (w1081:i64)  [unwired: 1 out]
              n684 = flat-sequence {
                tunnel: w1082 -> [w1109]
                tunnel: w1081 -> [w1108]
                tunnel: w1080 -> [w1087]
                tunnel: w1073 -> [w1090]
                tunnel: [w1090] -> w1078
                tunnel: [w1089] -> w1077
                tunnel: [w1086] -> w1076
                tunnel: [w1083] -> w1074
                tunnel: w1078 -> [w1145]
                tunnel: w1077 -> [w1143]
                tunnel: w1076 -> [w1142]
                tunnel: [w1141] -> w1075
                tunnel: w1074 -> [w1140]
                tunnel: [w1217] -> w1079
                tunnel: w1075 -> [w1216]
                frame #0 {
                  n685 = Divide(x=w1108, y=i64 1000) -> (x/y=w1103:dbl)
                  n686 = Multiply(x=w1103, y=w1109) -> (x*y=w1105:dbl)
                  n687 = local read "BD 1 Frequency 2 (MHz)"() -> (w1088:dbl)
                  n688 = Multiply(x="Osc. freq. (Hz)", y=6.283185307179586) -> (x*y=w1106:dbl)
                  n689 = Multiply(x=w1106, y=w1105) -> (x*y=w1085:dbl)
                  n690 = local read "BD 1 Frequency 1 (MHz)"() -> (w1093:dbl)
                  n691 = case shown="True" w1090 {
                    tunnel: w1085 -> [w1115 w1120]
                    tunnel: w1093 -> [_ w1131]
                    tunnel: w1088 -> [_ w1132]
                    tunnel: [w1112 w1126] -> w1091
                    tunnel: [FALSE w1123] -> w1086
                    tunnel: [0.0 w1116] -> w1083
                    frame False {
                      n692 = Sine(x=w1115) -> (sin(x)=w1113:dbl)
                      n693 = Multiply(x=w1113, y="Osc. amp. (MHz)") -> (x*y=w1112:dbl)
                    }
                    frame True {
                      n694 = Cosine(x=w1120) -> (cos(x)=w1135:dbl)
                      n695 = Subtract(x=w1132, y=w1131) -> (x-y=w1130:dbl)
                      n696 = Decrement(x=w1135) -> (x-1=w1134:dbl)
                      n697 = Subtract(x=w1130, y="Closest Delta (MHz)") -> (x-y=w1127:dbl)
                      n698 = Divide(x=w1134, y=-2.0) -> (x/y=w1128:dbl)
                      n699 = Multiply(x=w1128, y=w1127) -> (x*y=w1126:dbl)
                      n700 = local read "Vec Mean of T1 T2"() -> (w1122:dbl[])
                      n701 = Greater?(x=w1122, y="Stop F (pN)") -> (0:w1124:bool[])
                      n702 = Or Array Elements(Boolean array=w1124) -> (logical OR=w1123:bool)
                      n703 = Divide(x=w1120, y=6.283185307179586) -> (x/y=w1119:dbl)
                      n704 = Round Toward +Infinity(x=w1119) -> (ceil(x): smallest int >= x=w1116:dbl)
                      "Attempts" <- w1116
                      n705 = Greater?(x=w1116, y="Attempt Limit") -> (0:w1118:bool)
                      n706 = case shown="True" w1118 {
                        frame False {
                        }
                        frame True {
                          n707 = local write "Fish for Tether"(FALSE ("Fish for Tether")) -> ()
                          n708 = call <vilib>:"Beep.vi"() -> ()  [unwired: 3 in, 9 out]
                          n709 = local read "Messages"() -> (w1137:string)
                          n710 = call "Update messages.vi"("Message to add"="Tether fishing timeout." ("Messages"), "Old message string"=w1137) -> ("New message string"=→"Messages":string)
                        }
                      }
                    }
                  }
                  n711 = local read "BD 2 Frequency 1 (MHz)"() -> (w1092:dbl)
                  n712 = Select(t=w1093, s="Scan axis 2", f=w1092) -> (s? t:f=w1096:dbl)
                  n713 = Add(x=w1091, y=w1096) -> (x+y=w1089:dbl)
                  n714 = Select(t=w1089, s="Scan axis 2", f=w1093) -> (s? t:f=w1099:dbl)
                  n715 = Select(t=w1092, s="Scan axis 2", f=w1089) -> (s? t:f=w1098:dbl)
                  n716 = local read "Y RF Frequency Limits (MHz)"() -> (w1094:T16)
                  n717 = local read "X RF Frequency Limits (MHz)"() -> (w1095:T16)
                  n718 = local read "BD 1 Frequency 3 (MHz)"() -> (w1102:dbl)
                  n719 = local read "BD 2 Frequency 2 (MHz)"() -> (w1101:dbl)
                  n720 = local read "BD 2 Frequency 3 (MHz)"() -> (w1100:dbl)
                  n721 = call "set RF board frequency - interlace.vi"("Board 2 Frequency Limits"=w1094, "Board 1 Frequency Limits"=w1095, "FPGA VI Reference In"=w1087, "Board 2 Frequency 3 (MHz)"=w1100, "Board 1 Frequency 3 (MHz)"=w1102, "Board 2 Frequency 2 (MHz)"=w1101, "Board 2 Frequency 1 (MHz)"=w1098, "Board 1 Frequency 2 (MHz)"=w1088, "Board 1 Frequency 1  (MHz)"=w1099) -> ()  [unwired: 1 in, 2 out]
                }
                frame #1 {
                  n722 = And(x=w1145, y=w1142) -> (x .and. y?=w1144:bool)
                  n723 = case "Only if were fishing and now formed tether" shown="True" w1144 {
                    tunnel: w1143 -> [w1147 w1162]
                    tunnel: [w1146 w1161] -> w1141
                    tunnel: w1140 -> [_ w1157]
                    frame False {
                      n724 = local read "Fish for Tether"() -> (w1146:bool)
                      n725 = case shown="False" w1146 {
                        tunnel: w1147 -> [w1148 _]
                        frame False {
                          n726 = property on="BD 1 Frequency 1 (MHz)" class="DigNum (strict)"("Val(Sgnl)"=w1148) -> ()  [unwired: 2 in, 2 out]
                        }
                        frame True {
                        }
                      }
                    }
                    frame True {
                      w1161 = FALSE ("Fish for Tether")
                      n727 = call <vilib>:"Beep.vi"() -> ()  [unwired: 3 in, 9 out]
                      n728 = Number To Decimal String(number=w1157, width (-)=i16 1) -> (decimal integer string=w1155:string)
                      n729 = Concatenate Strings("Formed tether in ", w1155, " attempt(s)." ("string")) -> (w1152:string)
                      n730 = local read "Messages"() -> (w1159:string)
                      n731 = local write "Fish for Tether"(w1161) -> ()
                      n732 = call "Update messages.vi"("Message to add"=w1152, "Old message string"=w1159) -> ("New message string"=w1158:string)
                      n733 = local write "Messages"(w1158) -> ()
                      n734 = Get Date/Time In Seconds() -> (seconds since 1Jan1904=→"Time tether formed":timestamp)
                      n735 = local read "Flow ON during cal?"() -> (w1149:bool)
                      n736 = property on="Sample Channel\nFlow" class="Bool (strict)"("Val(Sgnl)"=w1149) -> (error out=w1150:errorcluster)  [unwired: 2 in, 1 out]
                      n737 = case shown="\"2\", \"3\", \"4\", \"5\", \"6\"" "Then..." {
                        selector: "Then..." -> [_ w1165]
                        tunnel: w1162 -> [w1164 _]
                        tunnel: w1150 -> [_ _]
                        frame "1", Default {
                          n738 = property on="BD 1 Frequency 1 (MHz)" class="DigNum (strict)"("Val(Sgnl)"=w1164) -> ()  [unwired: 2 in, 2 out]
                        }
                        frame "2", "3", "4", "5", "6" {
                          n739 = flat-sequence {
                            tunnel: w1165 -> [w1167]
                            frame #0 {
                              n740 = property on="Trap Delta (MHz)" class="DigNum (strict)"("Val(Sgnl)"="Move to Delta 1 (MHz)") -> ()  [unwired: 2 in, 2 out]
                            }
                            frame #1 {
                              n741 = case shown="\"5\", \"6\"" w1167 {
                                selector: w1167 -> [w1170 w1180 _]
                                frame "3", "4" {
                                n742 = flat-sequence {
                                tunnel: w1170 -> [w1171]
                                tunnel: [w1171] -> w1168
                                tunnel: [w1173] -> w1169
                                tunnel: w1168 -> [w1173]
                                tunnel: w1169 -> [w1177]
                                frame #0 {
                                n743 = property on="Green Laser ON/Interlacing" class="Bool (strict)"("Val(Sgnl)"=TRUE ("Value (Signaling)")) -> ()  [unwired: 2 in, 2 out]
                                }
                                frame #1 {
                                n744 = Multiply(x="Wait Before Save (s)", y=u32 1000 ("x")) -> (x*y=w1175:u32)
                                n745 = Wait (ms)(milliseconds to wait=w1175) -> ()  [unwired: 1 out]
                                }
                                frame #2 {
                                n746 = property on="Start Saving" class="Bool (strict)"("Value"=TRUE ("Start Saving")) -> ()  [unwired: 2 in, 2 out]
                                n747 = case shown="\"4\"" w1177 {
                                frame Default {
                                }
                                frame "4" {
                                n748 = property on="Fl. Triggered..." class="Bool (strict)"("Val(Sgnl)"=TRUE ("Value (Signaling)")) -> ()  [unwired: 2 in, 2 out]
                                }
                                }
                                }
                                }
                                }
                                frame "5", "6" {
                                n749 = stacked-sequence {
                                tunnel: w1180 -> [_ _ _ _ _ _ w1192]
                                frame #0 {
                                n750 = Replace Array Subset(array=u32[] [0] ("Index Values"), new element="Raster Set Upon Tether", index=0) -> (w1181:u32[])
                                n751 = property on="Saved AOD Raster Scan Parameter Sets" class="Arr (strict)"("Index Values"=w1181) -> ()  [unwired: 2 in, 2 out]
                                }
                                frame #1 {
                                n752 = Wait (ms)(milliseconds to wait=u32 500) -> ()  [unwired: 1 out]
                                }
                                frame #2 {
                                n753 = property on="Load parameters" class="Bool (strict)"("Val(Sgnl)"=TRUE ("Value (Signaling)")) -> ()  [unwired: 2 in, 2 out]
                                n754 = case shown="True" "Green ON During Raster" {
                                frame False {
                                }
                                frame True {
                                n755 = property on="Green Laser ON/Interlacing" class="Bool (strict)"("Val(Sgnl)"=TRUE ("Value (Signaling)")) -> ()  [unwired: 2 in, 2 out]
                                }
                                }
                                }
                                frame #3 {
                                n756 = Wait (ms)(milliseconds to wait=u32 500) -> ()  [unwired: 1 out]
                                }
                                frame #4 {
                                n757 = property on="Trap Raster Scan" class="Bool (strict)"("Val(Sgnl)"=TRUE ("Value (Signaling)")) -> ()  [unwired: 2 in, 2 out]
                                }
                                frame #5 {
                                n758 = Wait (ms)(milliseconds to wait=u32 2000) -> ()  [unwired: 1 out]
                                }
                                frame #6 {
                                n759 = flat-sequence {
                                tunnel: w1192 -> [w1199]
                                frame #0 {
                                n760 = while {
                                stop <- w1195 stop-if-true
                                n761 = local read "Raster Scanning..."() -> (w1194:bool)
                                n762 = local read "Saving..."() -> (w1197:bool)
                                n763 = Wait (ms)(milliseconds to wait=u32 100) -> ()  [unwired: 1 out]
                                n764 = Not(x=w1197) -> (.not. x?=w1196:bool)
                                n765 = Not(x=w1194) -> (.not. x?=w1193:bool)
                                n766 = And(x=w1196, y=w1193) -> (x .and. y?=w1195:bool)
                                }
                                }
                                frame #1 {
                                n767 = local read "Tether"() -> (w1200:bool)
                                n768 = case shown="True" w1200 {
                                tunnel: w1199 -> [_ w1202]
                                frame False {
                                n769 = property on="Fish for Tether" class="Bool (strict)"("Val(Sgnl)"="Fish again after \nraster break?") -> ()  [unwired: 2 in, 2 out]
                                }
                                frame True {
                                n770 = stacked-sequence {
                                tunnel: w1202 -> [_ w1206 _ _]
                                frame #0 {
                                n771 = property on="Trap Delta (MHz)" class="DigNum (strict)"("Val(Sgnl)"="Move to Delta 2 (MHz)") -> ()  [unwired: 2 in, 2 out]
                                n772 = case shown="True" "Flow ON after\ntether testing?" {
                                frame False {
                                }
                                frame True {
                                n773 = property on="Sample Channel\nFlow" class="Bool (strict)"("Val(Sgnl)"=TRUE ("Value (Signaling)")) -> ()  [unwired: 2 in, 2 out]
                                }
                                }
                                }
                                frame #1 {
                                n774 = flat-sequence {
                                tunnel: w1206 -> [w1208]
                                frame #0 {
                                n775 = Wait (ms)(milliseconds to wait=u32 500) -> ()  [unwired: 1 out]
                                }
                                frame #1 {
                                n776 = case shown="\"6\"" w1208 {
                                frame Default {
                                }
                                frame "6" {
